vi "Actor Core.vi"(8 "error in":errorcluster, 11 "Gui in":refnum<class "Gui.lvclass">) -> (0 "error out":errorcluster, 3 "Actor out":refnum<class "Actor.lvclass">)   [LabVIEW 2022 SP3, in "Test.lvlib" / "Gui.lvlib" / "Gui.lvclass"]
doc: "(<B>Filename</B>: Actor Framework.lvlib:Actor.lvclass:Actor Core.vi)\n\nReceives messages to the actor, reacts to them, and initiates any error handling that may shut the actor down.\n\nDescendant classes may override this VI to append parallel tasks for the actor to complete while it handles messages. Overrides use the Call Parent Class Method node."
uses:
  Gui.lvclass
  C:/Program Files (x86)/National Instruments/LabVIEW 2022/vi.lib/ActorFramework/Actor/Actor.lvclass
  <vilib>/ActorFramework/Actor/Actor.lvclass
  Gui.lvclass/Gui.ctl
  <vilib>/ActorFramework/Actor/Actor.lvclass/Actor.ctl
  <vilib>/ActorFramework/Message Enqueuer/Message Enqueuer.lvclass/Message Enqueuer.ctl
  <vilib>/ActorFramework/Message Enqueuer/Init from Existing Queue.vi
  <vilib>/ActorFramework/Message Enqueuer/Enqueue.vi
  <vilib>/ActorFramework/Stop Msg/Stop Msg.lvclass
  C:/Program Files (x86)/National Instruments/LabVIEW 2022/vi.lib/ActorFramework/Message/Message.lvclass
  <vilib>/ActorFramework/Message Priority Queue/Priority Enqueue.vi
  <vilib>/ActorFramework/Message Enqueuer/Message Enqueuer.lvclass
  LoggingActor/LoggingActor/LoggingActor.lvclass
panel:
  out "Uptime [s]":string
  # "<< Test GUI >>"
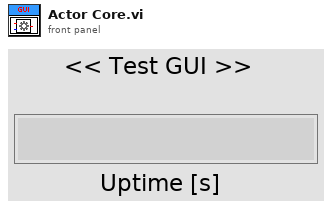
[diagram p1: front panel]
types:
  T1 = enum32{"Invalid", "Standard", "Closed", "Hidden", "Minimized", "Maximized"}
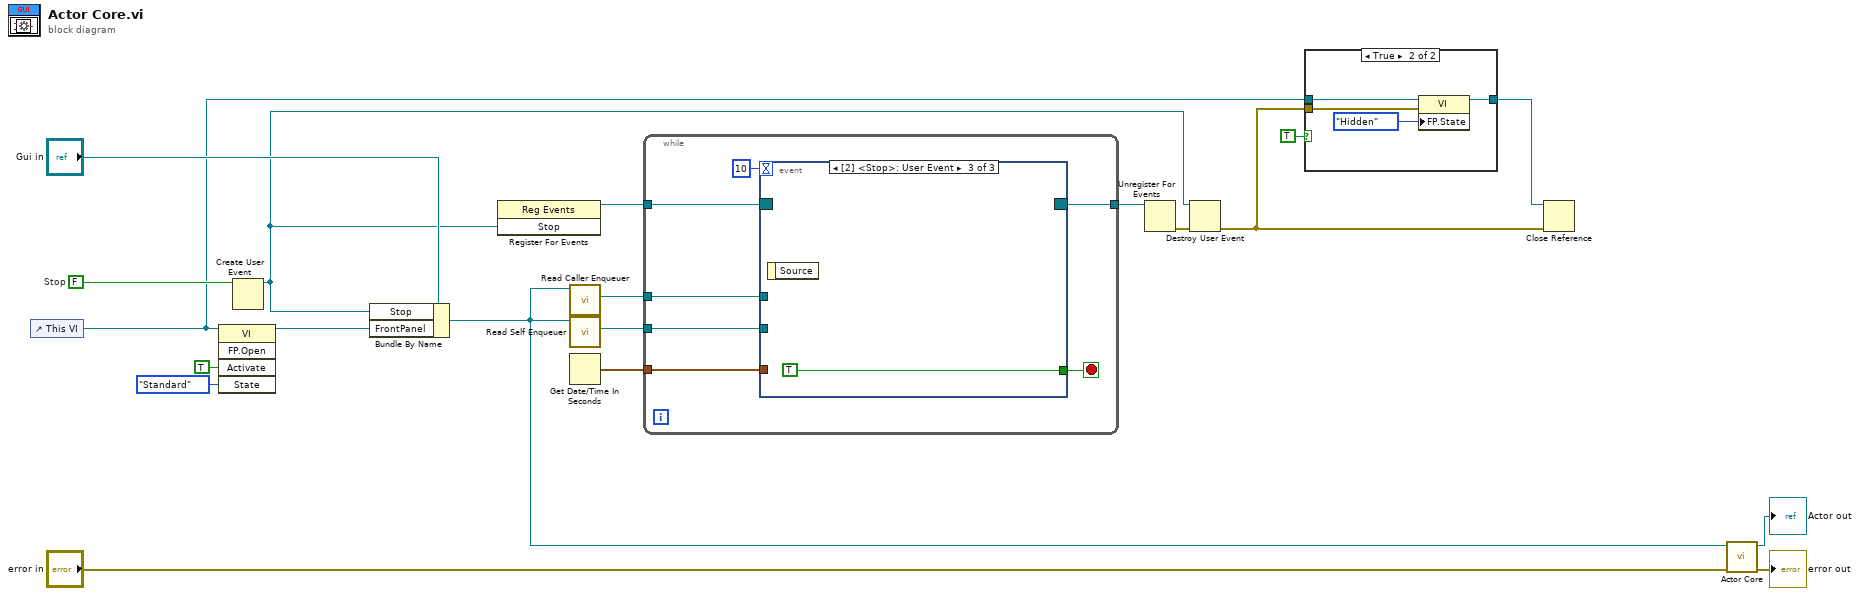
[diagram p0: block diagram]
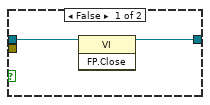
[diagram p2: hidden frame]
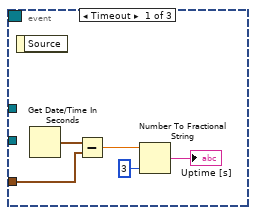
[diagram p3: hidden frame]
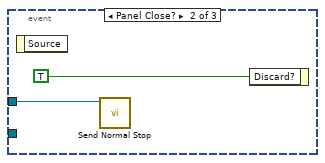
[diagram p4: hidden frame]
diagram:
  w12 = FALSE  # Stop
  n1 = control-ref of="This VI"() -> (w5:refnum<vi>)
  n2 = invoke class="VI" method="FP.Open"(reference=w5, "Activate"=TRUE ("Activate?"), "State"=T1."Standard") -> (reference out=w15:refnum<vi>)  [unwired: 2 in, 4 out]
  n3 = Create User Event(user event datatype=w12) -> (user event=w6:refnum<user-event>)  [unwired: 1 in, 1 out]
  n4 = Bundle By Name(cluster="Gui in", "Stop"=w6, "FrontPanel"=w15) -> (w16:refnum<class "Gui.lvclass">)
  n5 = register-events(w6) -> (reference out=w11:refnum<event-registration>)  [unwired: 2 in, 1 out]
  n6 = call <vilib>:"Read Caller Enqueuer.vi"("Actor"=w16) -> ("Caller Enqueuer"=w10:refnum<class "Message Enqueuer.lvclass">)  [unwired: 10 in]
  n7 = call <vilib>:"Read Self Enqueuer.vi"("Actor"=w16) -> ("Self Enqueuer"=w9:refnum<class "Message Enqueuer.lvclass">)  [unwired: 10 in]
  n8 = Get Date/Time In Seconds() -> (seconds since 1Jan1904=w4:timestamp)
  n9 = while {
    tunnel: w11 -> [w26]
    tunnel: w10 -> [w25]
    tunnel: w9 -> [w24]
    tunnel: [w23] -> w8
    tunnel: w4 -> [w21]
    stop <- w27 stop-if-true
    n10 = event shown="[2] <Stop>: User Event" {
      selector: w26 -> [_ _ _]
      dyn-events: [_ _ _] -> w23
      timeout: 10 -> [_ _ _]
      tunnel: [_ _ TRUE ("Discard?")] -> w27
      tunnel: w25 -> [_ w33 _]
      tunnel: w24 -> [_ _ _]
      tunnel: w21 -> [w31 _ _]
      event Timeout {
        n11 = event-data() -> ()  [unwired: 1 in, 1 out]
        n12 = Get Date/Time In Seconds() -> (seconds since 1Jan1904=w32:timestamp)
        n13 = Subtract(x=w32, y=w31) -> (x-y=w30:dbl)
        n14 = Number To Fractional String(number=w30, precision (6)=i16 3) -> (F-format string=→"Uptime [s]":string)  [unwired: 2 in]
      }
      event Panel Close? {
        n15 = event-data() -> ()  [unwired: 1 in, 1 out]
        n16 = call <vilib>:"Send Normal Stop.vi"("Message Enqueuer"=w33) -> ()  [unwired: 10 in, 1 out]
        n17 = event-data("Discard?"=TRUE) -> ()  [unwired: 1 in, 1 out]
      }
      event User Event {
        n18 = event-data() -> ()  [unwired: 1 in, 1 out]
      }
    }
  }
  n19 = Unregister For Events(event registration refnum=w8) -> (error out=w7:errorcluster)  [unwired: 1 in]
  n20 = Destroy User Event(user event=w6, error in=w7) -> (error out=w2:errorcluster)
  n21 = case shown="True" TRUE {
    tunnel: w5 -> [w37 w41]
    tunnel: [w36 w40] -> w3
    tunnel: w2 -> [_ w39]
    frame False {
      n22 = invoke class="VI" method="FP.Close"(reference=w37) -> (reference out=w36:refnum<vi>)  [unwired: 2 in, 2 out]
    }
    frame True {
      n23 = property class="VI"(reference=w41, error in=w39, "FP.State"=T1."Hidden" ("Front Panel Window:State")) -> (reference out=w40:refnum<vi>)  [unwired: 1 out]
    }
  }
  n24 = Close Reference(reference=w3, error in (no error)=w2) -> ()  [unwired: 1 out]
  n25 = call-parent "Actor Core.vi"("error in"="error in", "Actor in"=w16) -> ("error out"=→"error out":errorcluster, "Actor out"=→"Actor out":refnum<class "Actor.lvclass">)  [unwired: 8 in]
